vi "magnet_to_position.vi"(3 "magetic field":T1) -> (1 "normalized position":T1)   [LabVIEW 2017]
uses:
  typedefs/reading3.ctl
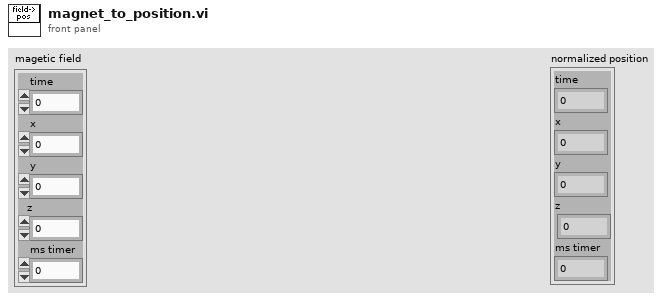
[diagram p1: front panel]
types:
  T1 = typedef "reading3.ctl" = cluster{"time":dbl, "x":dbl, "y":dbl, "z":dbl, "ms timer":u32}
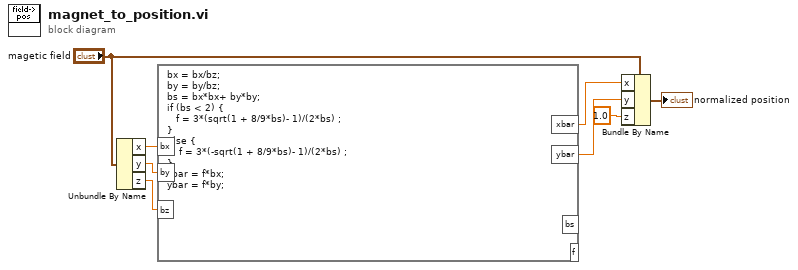
[diagram p0: block diagram]
diagram:
  n1 = Unbundle By Name("magetic field") -> ("x"=w8:dbl, "y"=w7:dbl, "z"=w6:dbl)
  n2 = formula code="bx = bx/bz;\nby = by/bz;\nbs = bx*bx+ by*by;\nif (bs < 2) {\n   f = 3*(sqrt(1 + 8/9*bs)- 1)/(2*bs) ;\n} \nelse {\n    f = 3*(-sqrt(1 + 8/9*bs)- 1)/(2*bs) ;\n}\nxbar = f*bx; \nybar = f*by;"("bx"=w8, "by"=w7, "bz"=w6) -> ("xbar"=w3:dbl, "ybar"=w2:dbl)  [unwired: 2 out]
  n3 = Bundle By Name(cluster="magetic field", "x"=w3, "y"=w2, "z"=1.0) -> (→"normalized position":T1)
